vi "Work.vi"(0 "Action":T2, 5 "Init":T3={"Sample Frequency"=1000.0, "Sample Count"=1000.0} {"Sample Frequency" format="%.2p"}, 7 "Tag":T4={"Shape"=enum."Sine", "Frequency"=1000.0, "Amplitude"=1.0, "Phase"=0.0, "Offset"=0.0}, 12 "State in":T1) -> (4 "Out":cluster{"t0":dbl, "dt":dbl, "y":dbl[]}, 14 "State out":T1, 15 "Error":errorcluster)   [LabVIEW 2020, in "Function Generator.lvlib"]
uses:
  Function Generator.lvlib
  Tags.ctl
  Block/FlexBlocks/Shape.ctl
  Init.ctl
  Block/FlexBlocks/Worker Action.ctl
  State.ctl
  <vilib>/measure/NI_MABase.lvlib
  Block/FlexBlocks/FlexBlocks.lvlib
panel:
  # "Indicators on the connector pane will be put into a FlexChannel behind the scenes to publish the values to other blocks and user code."
  # "Anything in a cluster named Init will be set once by FlexBlocks and remain static for all iterations."
  # "Controls in a cluster named Tags will be broken out into separate FlexChannels and read with the latest value endpoint to be passed into the block."
  # "\"State in\" and \"State out\" are also special names that the framework will maintain for the worker and pass the previous call's State out value to State in. During the Init call, State in will use default values, not the default values applied on the VI."
  # "Usage of State terminals is optional and if the VI is set to Preallocated Reentrancy, feedback nodes can be used instead."
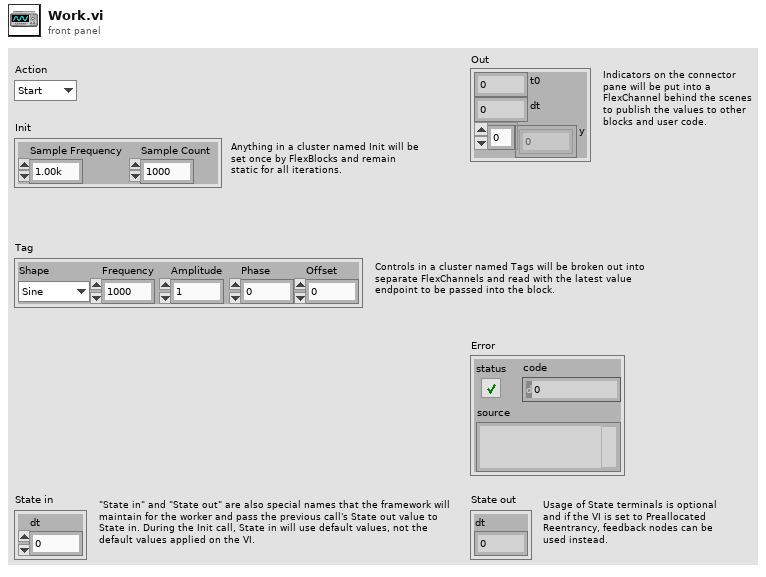
[diagram p1: front panel]
types:
  T1 = typedef "Function Generator.lvlib/State.ctl" = cluster{"dt":dbl}
  T2 = typedef "FlexBlocks.lvlib/Worker Action.ctl" = enum16{"Start", "Work", "Stop"}
  T3 = typedef "Function Generator.lvlib/Init.ctl" = cluster{"Sample Frequency":dbl, "Sample Count":dbl}
  T4 = typedef "Function Generator.lvlib/Tags.ctl" = cluster{"Shape":T5, "Frequency":dbl, "Amplitude":dbl, "Phase":dbl, "Offset":dbl}
  T5 = typedef "Function Generator.lvlib/Shape.ctl" = enum16{"Sine", "Square", "Triangle", "Saw"}
  T6 = enum16{"Sine Wave", "Triangle Wave", "Square Wave", "Sawtooth Wave"}
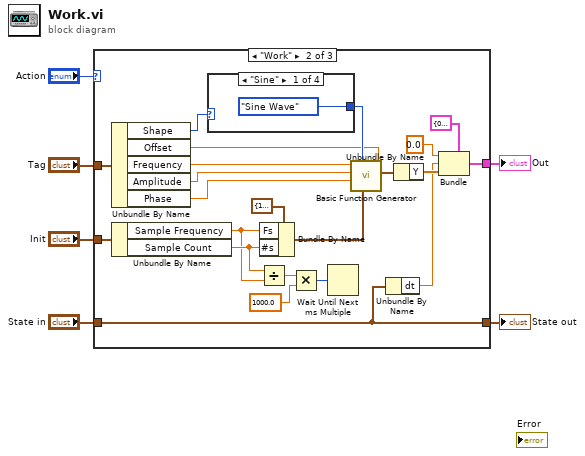
[diagram p0: block diagram]
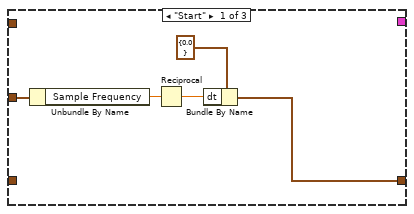
[diagram p2: hidden frame]
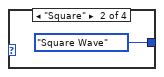
[diagram p3: hidden frame]
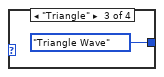
[diagram p4: hidden frame]
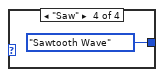
[diagram p5: hidden frame]
diagram:
  n1 = case shown="\"Work\"" "Action" {
    tunnel: "Init" -> [w11 w29 _]
    tunnel: "Tag" -> [_ w33 _]
    tunnel: [_ w19 _] -> w3
    tunnel: "State in" -> [_ w18 w38]
    tunnel: [w8 w18 w38] -> w1
    frame "Start" {
      n2 = Unbundle By Name(w11) -> ("Sample Frequency"=w10:dbl)
      n3 = Reciprocal(x=w10) -> (1/x=w7:dbl)
      n4 = Bundle By Name(cluster=T1 {"dt"=0.0} ("State in"), "dt"=w7) -> (w8:T1)
    }
    frame "Work" {
      n5 = Unbundle By Name(w33) -> ("Shape"=w32:T5, "Offset"=w26:dbl, "Frequency"=w30:dbl, "Amplitude"=w28:dbl, "Phase"=w27:dbl)
      n6 = Unbundle By Name(w29) -> ("Sample Frequency"=w15:dbl, "Sample Count"=w16:dbl)
      n7 = case shown="\"Sine\"" w32 {
        tunnel: [T6."Sine Wave" ("signal type") T6."Square Wave" ("signal type") T6."Triangle Wave" ("signal type") T6."Sawtooth Wave" ("signal type")] -> w31
        frame "Sine" {
        }
        frame "Square" {
        }
        frame "Triangle" {
        }
        frame "Saw" {
        }
      }
      n8 = Divide(x=w16, y=w15) -> (x/y=w14:dbl)
      n9 = Bundle By Name(cluster=cluster{"Fs":dbl, "#s":dbl} {"Fs"=1000.0, "#s"=1000.0} ("sampling info"), "Fs"=w15, "#s"=w16) -> (w24:cluster{"Fs":dbl, "#s":dbl})
      n10 = Multiply(x=w14, y=1000.0) -> (x*y=w12:u32)
      n11 = Wait Until Next ms Multiple(millisecond multiple=w12) -> ()  [unwired: 1 out]
      n12 = call <vilib>:"Basic Function Generator.vi"("offset"=w26, "sampling info"=w24, "signal type"=w31, "phase"=w27, "amplitude"=w28, "frequency"=w30) -> ("signal out"=w23:waveform(dbl))  [unwired: 3 in, 2 out]
      n13 = Unbundle By Name(w18) -> ("dt"=w17:dbl)
      n14 = Unbundle By Name(w23) -> ("Y"=w22:dbl[])
      n15 = Bundle(cluster=cluster{"t0":dbl, "dt":dbl, "y":dbl[]} {"t0"=0.0, "dt"=0.0, "y"=[]}, "t0"=0.0, "dt"=w17, "y"=w22) -> (w19:cluster{"t0":dbl, "dt":dbl, "y":dbl[]})
    }
    frame "Stop" {
    }
  }
  "Out" <- w3
  "State out" <- w1
